vi "(FPGA)_PIDXYZ_laserPID)_COMtemp2.vi"() -> ()   [LabVIEW 2018]
doc: "This VI will read single point values from 4 channels of a R Series board at a specified rate."
uses:
  <vilib>/rvi/Emulation/niFpgaGetClockAttributes.vi
  <vilib>/rvi/Emulation/niFpgaSctlEmulationGetInTimedLoop.vi
  <vilib>/rvi/Emulation/niFpgaEmulationReportErrorSimple.vi
  <vilib>/rvi/eio/common/nirviEmuTemplateMethod_errors.vi
  <vilib>/rvi/Emulation/niFpgaProcessEmulError.vi
  <vilib>/rvi/Emulation/niFpgaCriticalErrorInLSC.vi
  <vilib>/rvi/Memory/Memory_Emulation/nirvimemoryFastEmulation.vi
  <vilib>/rvi/Memory/Memory_Emulation/nirvimemoryEmulation.vi
  <vilib>/rvi/Emulation/niFpgaEmulationIsFPGAContextNoSignature.vi
  <vilib>/rvi/DataTransferAndStorage/Container/Common/niFpgaContainerGetUniqueNameForEmu.vi
  <vilib>/rvi/errors/nirviReportUnexpectedCaseInternalError (U32).vi
  <vilib>/rvi/Memory/Memory_Emulation/niFpgaMemoryEmulationCacheClearOnFirstRun.vi
  <vilib>/rvi/Memory/Memory_Emulation/nirvimemoryEmulationManagerCache_MakeExclusive.vi
  <vilib>/rvi/Memory/Memory_Emulation/niFpgaMemoryEmulationValidateCache.vi
  <vilib>/rvi/Memory/Memory_Emulation/nirvimemoryEmulationManagerCache_InsertValue.vi
  <vilib>/Utility/error.llb/Clear Errors.vi
  <vilib>/rvi/Memory/Memory_Emulation/nirvimemoryEmulationManagerCache_ReleaseExclusive.vi
  <vilib>/rvi/Memory/Memory_Emulation/nirvimemoryEmulationManagerCache_GetValue.vi
  <vilib>/rvi/Memory/Memory_Emulation/nirvimemoryEmulationManagerCache_SetValue.vi
  <vilib>/rvi/Emulation/niFpgaSctlEmulationResourceMgr.vi
  <vilib>/eio/EIONode/EIONode.xnode
  <vilib>/rvi/DataTransferAndStorage/Container/XNode/niFpgaContainer.xnode
  <vilib>/rvi/FXPMathLib/FxpInterpret/XNode/nifxpmath_Interpret.xnode
panel:
  out "accum out z2":fxp<+/-,37,37>
  out "accurm reset z2":bool
  out "accum out z1":fxp<+/-,37,37>
  out "accum reset z1":bool
  in  "Reset x accum":bool
  in  "Reset y accum":bool
  in  "Reset z accum":bool
  out "master y":bool
  out "master x":bool
  in  "No_integral_gain":bool=TRUE
  in  "Y_emergency_threshould":i16
  in  "X_emergency_threshould":i16
  in  "Big Number":sgl
  in  "Amplitude_sine_EOM":sgl
  in  "eom sine frequency (periods/tick)":fxp<+,32,0>=0.0002500000409781933
  in  "pz?":bool
  out "pg Z mod":fxp<+/-,24,12>
  in  "pg Z":fxp<+/-,24,12>
  in  "amplitude":i16=8192
  in  "offset":i16=8192
  out "Trigger for COM out":i16 caption="square wave out"
  out "dgz mod":fxp<+/-,24,12>
  in  "activate COMz":bool
  in  "dg Z":fxp<+/-,24,12>
  in  "activate COMy":bool
  out "dgy mod":fxp<+/-,24,12>
  in  "dg Y":fxp<+/-,24,12>
  out "dgx mod":fxp<+/-,24,12>
  in  "activate COMx":bool
  in  "dg X":fxp<+/-,24,12>
  in  "duty cycle (periods)":fxp<+,32,0>=0.5
  in  "frequency (periods/tick)":fxp<+,32,0>=0.00390625
  in  "final filter coeff X before":i32[](array[numeric])=[-955995012, 2025731616, 1001305, -1023351008, 2092954700, 1034533]
  in  "final filter coeff X":i32[](array[numeric])=[-955995012, 2025731616, 1001305, -1023351008, 2092954700, 1034533]
  in  "final filter coeff Y before":i32[](array[numeric])=[-955995012, 2025731616, 1001305, -1023351008, 2092954700, 1034533]
  in  "final filter coeff Y":i32[](array[numeric])=[-955995012, 2025731616, 1001305, -1023351008, 2092954700, 1034533]
  in  "final filter coeff Z":i32[](array[numeric])=[-955995012, 2025731616, 1001305, -1023351008, 2092954700, 1034533]
  in  "final filter coeff Z before":i32[](array[numeric])=[-955995012, 2025731616, 1001305, -1023351008, 2092954700, 1034533]
  in  "LP Coeff Z before":i32[](array[numeric])=[1008310688, 32715568]
  in  "LP Coeff Z":i32[](array[numeric])=[1008310688, 32715568]
  in  "LP Coeff X":i32[](array[numeric])=[1008310688, 32715568]
  in  "LP Coeff X before":i32[](array[numeric])=[1008310688, 32715568]
  in  "LP Coeff Y before":i32[](array[numeric])=[1008310688, 32715568]
  in  "LP Coeff Y":i32[](array[numeric])=[1008310688, 32715568]
  in  "Upper lim Z before":fxp<+/-,16,16>
  in  "Lower lim Z before":fxp<+/-,16,16>
  in  "Upper lim Y before":fxp<+/-,16,16>
  in  "Lower lim Y before":fxp<+/-,16,16>
  in  "Upper lim X before":fxp<+/-,16,16>
  in  "Lower lim X before":fxp<+/-,16,16>
  in  "HP coeff band X before":i32[](array[numeric])=[-850883994, 1909449570, 958518847, -975456236, 2033039520, 1020559395]
  in  "LP Coeff band X before":i32[](array[numeric])=[-955995012, 2025731616, 1001305, -1023351008, 2092954700, 1034533]
  in  "LP Coeff band X":i32[](array[numeric])=[-955995012, 2025731616, 1001305, -1023351008, 2092954700, 1034533]
  in  "HP Coeff band X":i32[](array[numeric])=[-850883994, 1909449570, 958518847, -975456236, 2033039520, 1020559395]
  in  "dg band X before":fxp<+/-,24,12>
  in  "dg band X":fxp<+/-,24,12>
  in  "HP Coeff X before":i32[](array[numeric])=[946630756, 1010186290]
  in  "HP Coeff X":i32[](array[numeric])=[946630756, 1010186290]
  in  "Use X PID before":bool
  out "AI X before chamber plot":i16
  in  "X before Setpoint":i16
  out "tot_fb X plot":i16
  out "fb X before chamber plot":i16
  in  "DC offset X":i16
  in  "pg X before":fxp<+/-,24,12>
  in  "ig X before":fxp<+/-,24,-4>
  in  "dg X before":fxp<+/-,24,12>
  out "fb X plot":i16
  in  "ig X":fxp<+/-,24,-4>
  in  "Lower lim X":fxp<+/-,16,16>
  in  "Upper lim X":fxp<+/-,16,16>
  in  "pg X":fxp<+/-,24,12>
  out "AI X plot":i16
  in  "X Setpoint":i16
  in  "HP coeff band Y before":i32[](array[numeric])=[-850883994, 1909449570, 958518847, -975456236, 2033039520, 1020559395]
  in  "LP Coeff band Y before":i32[](array[numeric])=[-955995012, 2025731616, 1001305, -1023351008, 2092954700, 1034533]
  in  "LP Coeff band Y":i32[](array[numeric])=[-955995012, 2025731616, 1001305, -1023351008, 2092954700, 1034533]
  in  "HP Coeff band Y":i32[](array[numeric])=[-850883994, 1909449570, 958518847, -975456236, 2033039520, 1020559395]
  in  "dg band Y before":fxp<+/-,24,12>
  in  "dg band Y":fxp<+/-,24,12>
  in  "HP Coeff Y before":i32[](array[numeric])=[946630756, 1010186290]
  in  "HP Coeff Y":i32[](array[numeric])=[946630756, 1010186290]
  in  "Use Y PID before":bool
  out "AI Y before chamber plot":i16
  in  "Y before Setpoint":i16
  out "tot_fb Y plot":i16
  out "fb Y before chamber plot":i16
  in  "DC offset Y":i16
  in  "pg Y before":fxp<+/-,24,12>
  in  "ig Y before":fxp<+/-,24,-4>
  in  "dg Y before":fxp<+/-,24,12>
  out "fb Y plot":i16
  in  "ig Y":fxp<+/-,24,-4>
  in  "Lower lim Y":fxp<+/-,16,16>
  in  "Upper lim Y":fxp<+/-,16,16>
  in  "pg Y":fxp<+/-,24,12>
  out "AI Y plot":i16
  in  "Y Setpoint":i16
  in  "EOM_offset":i16
  in  "EOM_seed":u32=4294967295 caption="seed"
  in  "EOM reset":bool caption="reset"
  in  "EOM_threshold":i16
  in  "EOM_amplitude":i16
  in  "HP coeff band Z before":i32[](array[numeric])=[-850883994, 1909449570, 958518847, -975456236, 2033039520, 1020559395]
  in  "LP Coeff band Z before":i32[](array[numeric])=[-955995012, 2025731616, 1001305, -1023351008, 2092954700, 1034533]
  in  "LP Coeff band Z":i32[](array[numeric])=[-955995012, 2025731616, 1001305, -1023351008, 2092954700, 1034533]
  in  "HP Coeff band Z":i32[](array[numeric])=[-850883994, 1909449570, 958518847, -975456236, 2033039520, 1020559395]
  in  "dg band Z before":fxp<+/-,24,12>
  in  "dg band Z":fxp<+/-,24,12>
  in  "data_buffer3":i16
  in  "Arb gain (ch2)":fxp<+/-,24,12>=0.5 caption="RMS"
  in  "HP Coeff Z before":i32[](array[numeric])=[946630756, 1010186290]
  in  "HP Coeff Z":i32[](array[numeric])=[946630756, 1010186290]
  in  "Use Z PID before":bool
  out "AI Z before chamber plot":i16
  in  "Z before Setpoint":i16
  out "tot_fb Z plot":i16
  out "fb Z before chamber plot":i16
  in  "DC offset Z":i16
  in  "pg Z before":fxp<+/-,24,12>
  in  "ig Z before":fxp<+/-,24,-4>
  in  "dg Z before":fxp<+/-,24,12>
  out "fb Z plot":i16
  in  "ig Z":fxp<+/-,24,-4>
  out "written_address":u32
  in  "ready_to_write":bool
  in  "Arb steps per cycle":u16
  in  "data_buffer2":i16
  in  "data_buffer_1":i16
  in  "write_address":u16
  in  "Arb gain (ch1)":fxp<+/-,24,12>=0.5 caption="RMS"
  in  "Arb gain (ch0)":fxp<+/-,24,12>=0.5 caption="RMS"
  in  "Lower lim Z":fxp<+/-,16,16>
  in  "Upper lim Z":fxp<+/-,16,16>
  out "AI Z plot":i16
  in  "Z Setpoint":i16
  in  "Count(uSec)":u32
  out "FPGA Error Out":errorcluster
  in  "Stop":bool
  # "test"
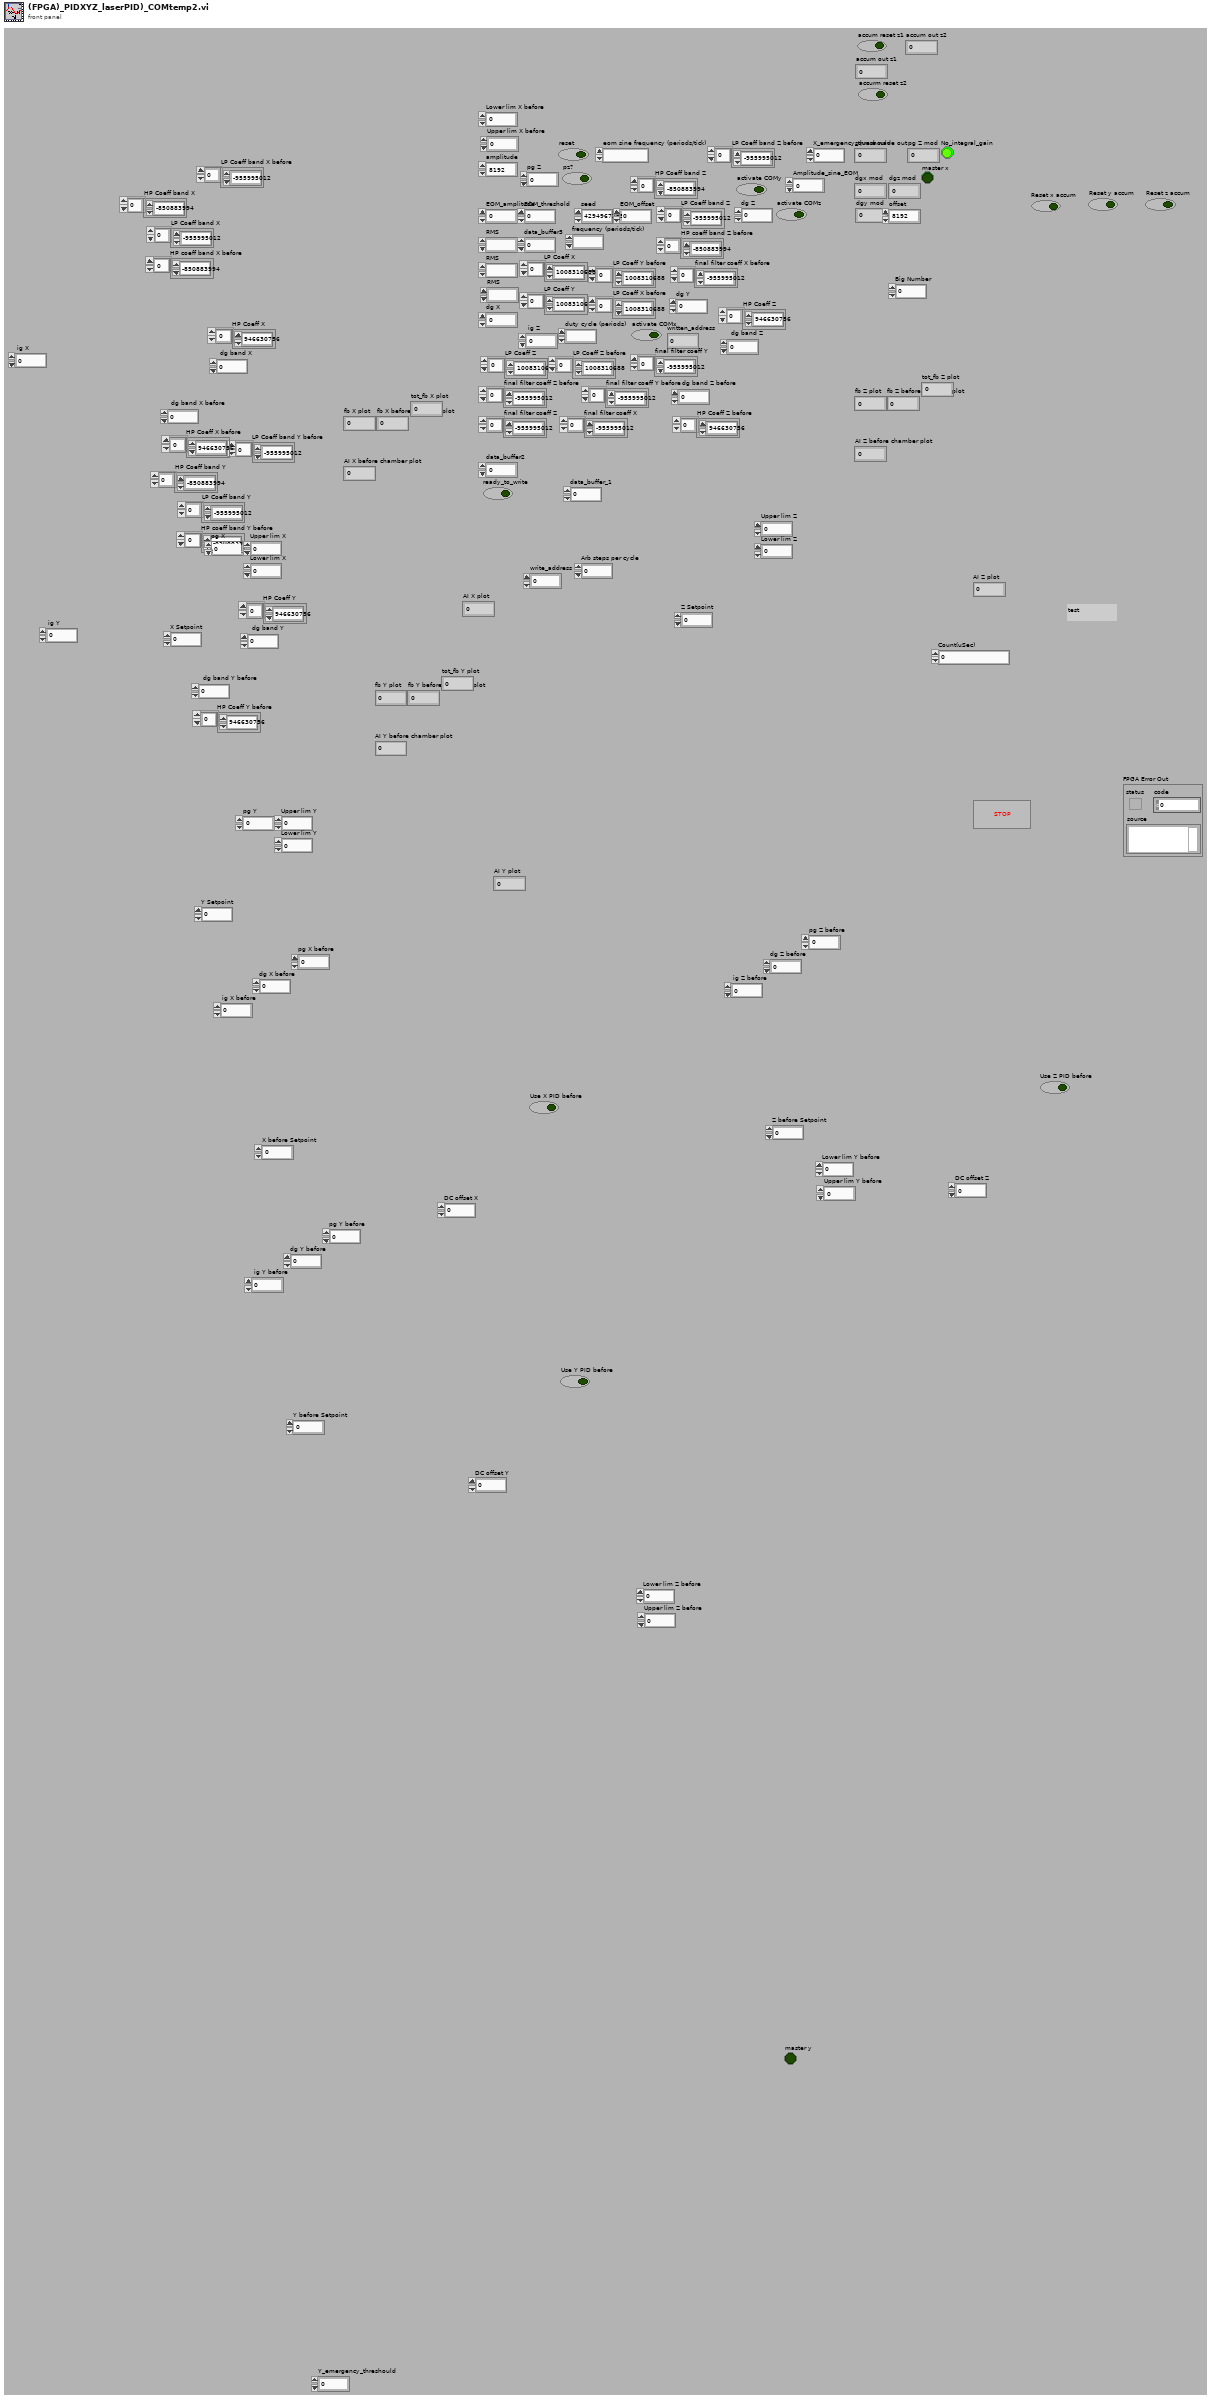
[diagram p1: front panel]
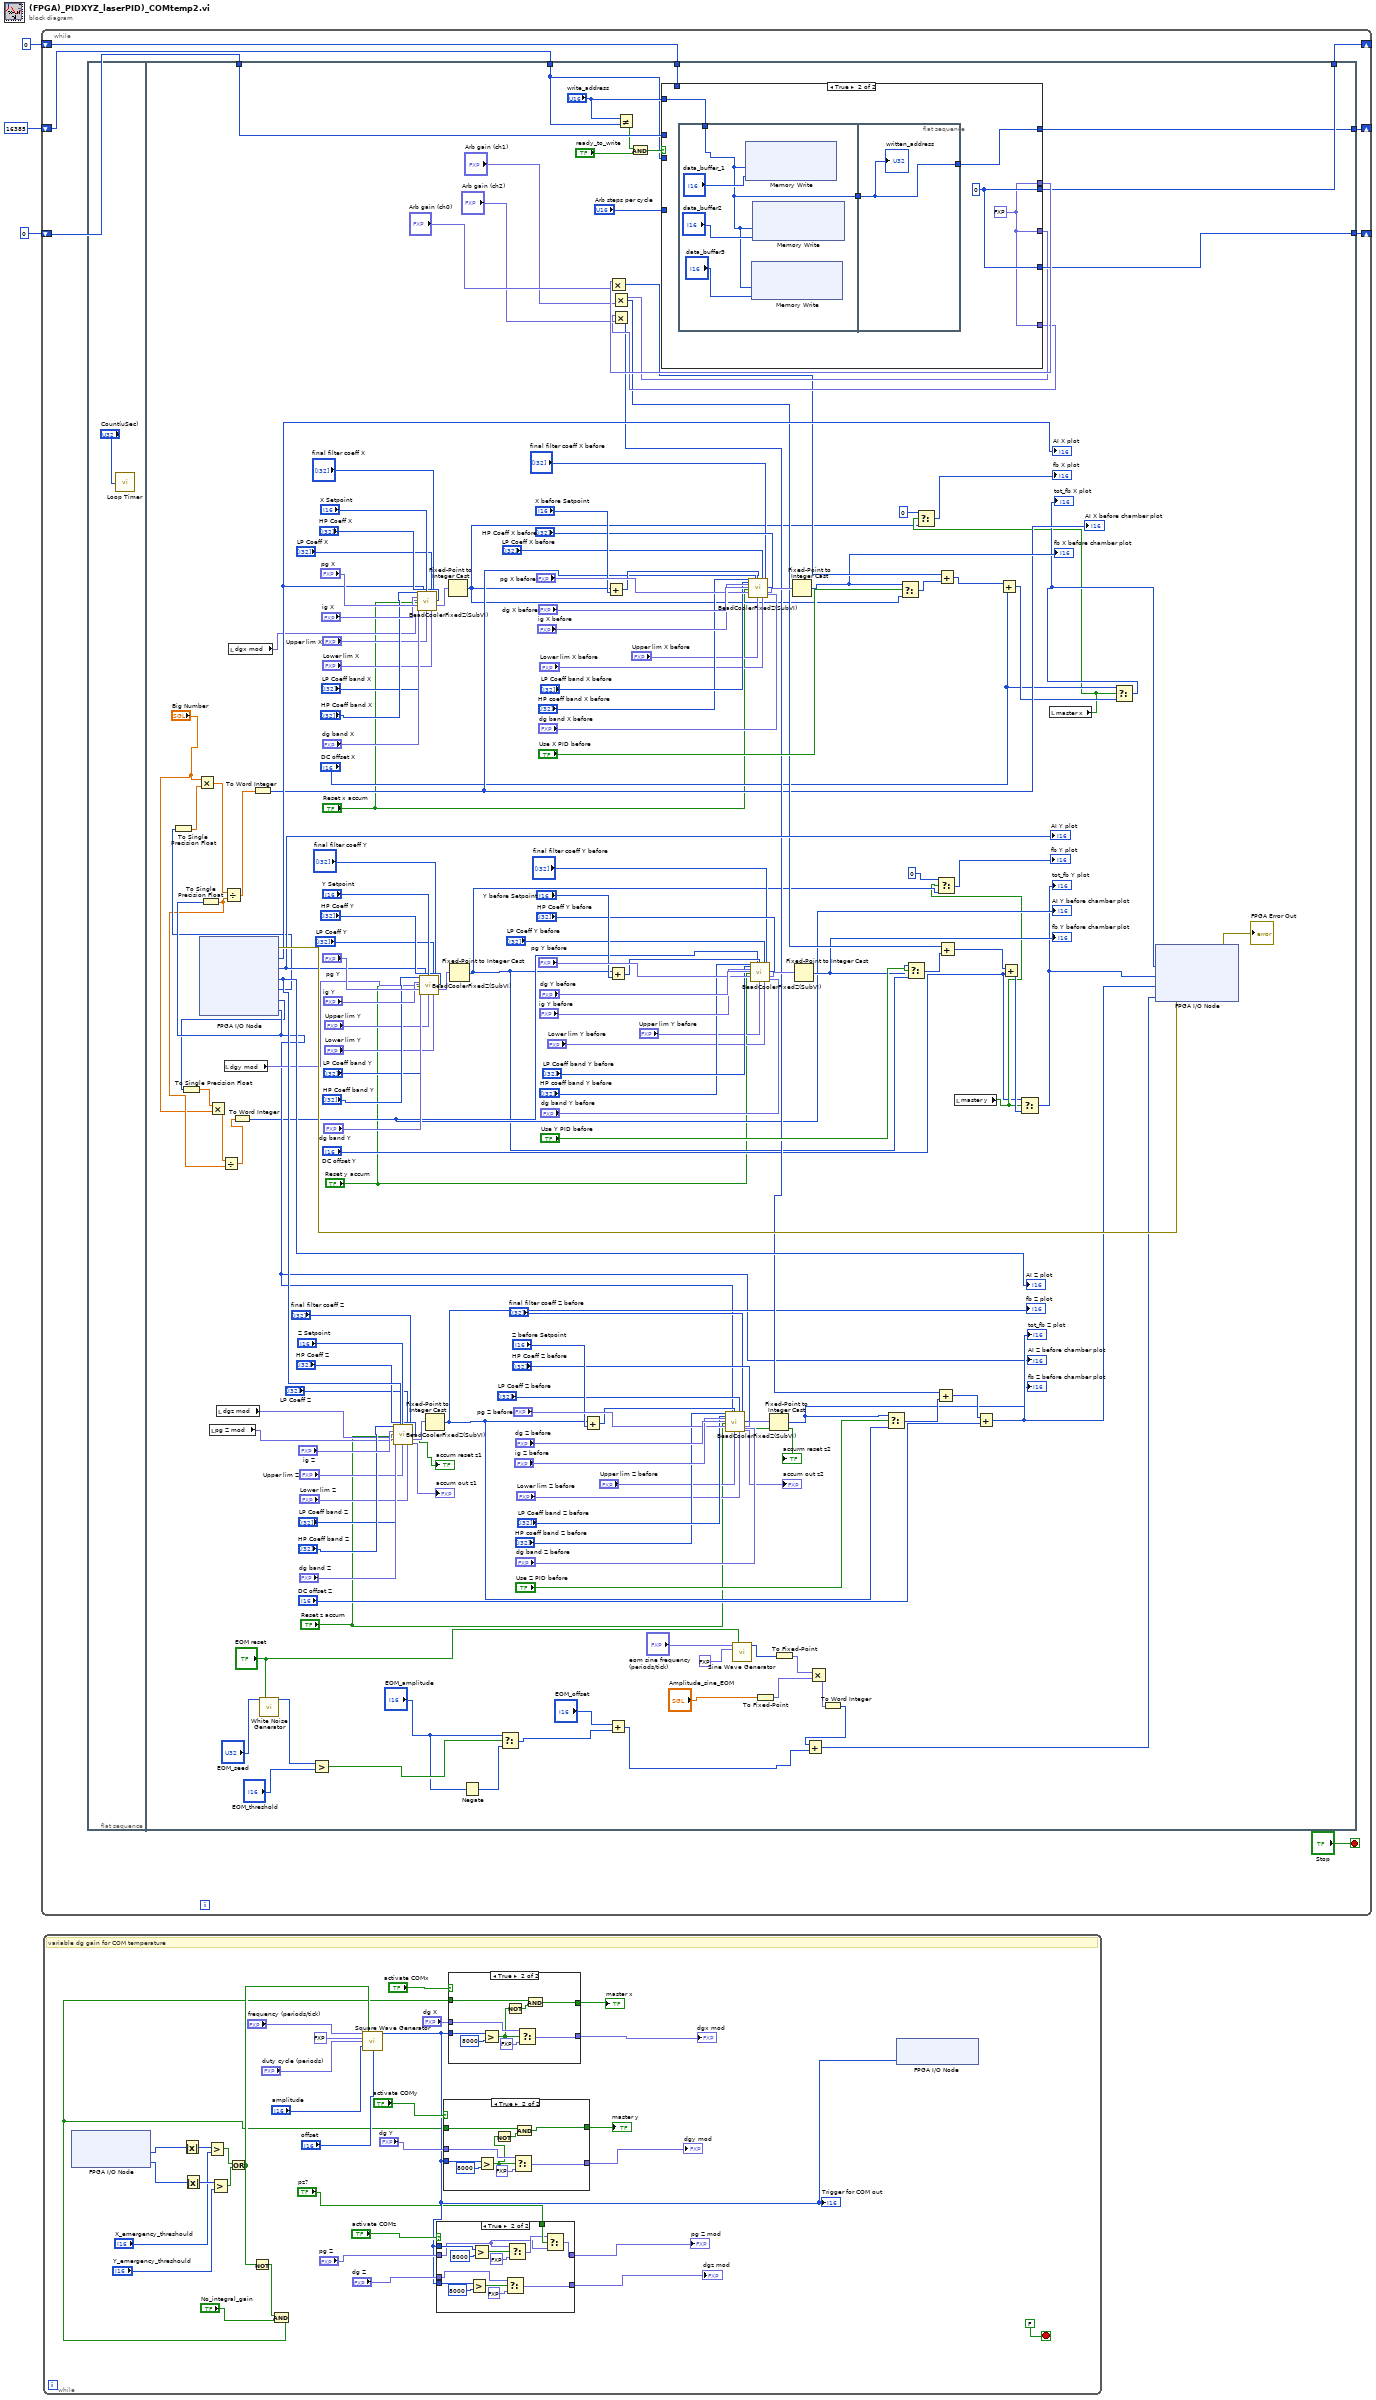
[diagram p0: block diagram]
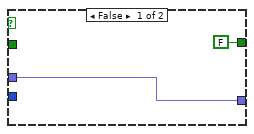
[diagram p3: hidden frame]
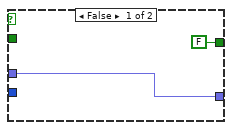
[diagram p4: hidden frame]
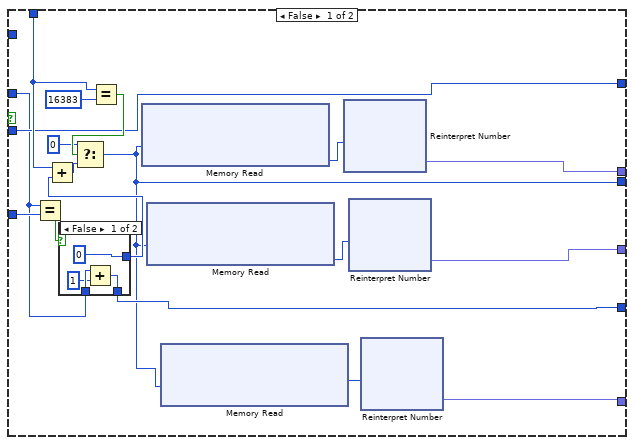
[diagram p5: hidden frame]
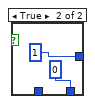
[diagram p6: hidden frame]
diagram:
  n1 = while {
    shift-right: [w9] -> _
    shift-left: u16 0 ("t") -> [w8]
    shift-right: [w7] -> _
    shift-left: u16 0 ("t") -> [w4]
    shift-right: [w6] -> _
    shift-left: u32 16385 ("write_address") -> [w5]
    stop <- "Stop" stop-if-true
    n2 = flat-sequence {
      tunnel: [w180] -> w9
      tunnel: w8 -> [w179]
      tunnel: [w177] -> w7
      tunnel: w4 -> [w176]
      tunnel: [w175] -> w6
      tunnel: w5 -> [w168]
      frame #0 {
        n3 = call "Loop Timer"("Count(uSec)"="Count(uSec)") -> ()  [unwired: 1 out]
      }
      frame #1 {
        n4 = xnode "FPGA I/O Node"() -> ("error out"=w185:errorcluster, "Connector0/AI0"=w92:i16, "Connector0/AI1"=w114:i16, "Connector0/AI2"=w166:i16, "Connector0/AI3"=w40:i16, "Connector0/AI4"=w39:i16, "Connector0/AI5"=w44:i16)  [unwired: 7 in, 6 out]
        "AI Z plot" <- w166
        "AI Z before chamber plot" <- w44
        "AI Y plot" <- w114
        "AI X plot" <- w92
        n5 = To Single Precision Float(number=w40) -> (single precision float=w43:sgl)
        n6 = To Single Precision Float(number=w39) -> (single precision float=w38:sgl)
        n7 = Multiply(x="Big Number", y=w43) -> (x*y=w42:sgl)
        n8 = To Single Precision Float(number=w44) -> (single precision float=w36:sgl)
        n9 = Multiply(x=w38, y="Big Number") -> (x*y=w37:sgl)
        n10 = local read "pg Z mod"() -> (w57:fxp<+/-,24,12>)
        n11 = local read "dgz mod"() -> (w58:fxp<+/-,24,12>)
        n12 = Divide(x=w37, y=w36) -> (x/y=w35:sgl)
        n13 = Divide(x=w42, y=w36) -> (x/y=w41:sgl)
        n14 = local read "dgy mod"() -> (w59:fxp<+/-,24,12>)
        n15 = local read "dgx mod"() -> (w60:fxp<+/-,24,12>)
        n16 = To Word Integer(number=w35) -> (16bit integer=w34:i16)
        "AI Y before chamber plot" <- w34
        n17 = To Word Integer(number=w41) -> (16bit integer=w45:i16)
        "AI X before chamber plot" <- w45
        n18 = call "White Noise Generator"("seed"="EOM_seed", "reset"="EOM reset") -> ("white noise out"=w145:i16)  [unwired: 13 in]
        n19 = Greater?(x=w145, y="EOM_threshold") -> (0:w143:bool)
        n20 = call "BeadCoolerFixedZ(SubVI).vi"("hp coeff band"="HP Coeff band Z", "lp coeff band"="LP Coeff band Z", "ig"="ig Z", "dg"=w58, "load (F)"="Reset z accum", "pg"=w57, "dg band"="dg band Z", "AI0"=w166, "Dc Pos"="Z Setpoint", "Upper lim"="Upper lim Z", "lp coeff"="LP Coeff Z", "Lower lim"="Lower lim Z", "final filter coeff"="final filter coeff Z", "hp coeff"="HP Coeff Z") -> ("Output"=w155:fxp<+/-,16,16>, "accurm reset"=→"accum reset z1":bool, "accum out"=→"accum out z1":fxp<+/-,37,37>)  [unwired: 11 in]
        n21 = call "BeadCoolerFixedZ(SubVI).vi"("hp coeff band"="HP Coeff band X", "lp coeff band"="LP Coeff band X", "ig"="ig X", "dg"=w60, "load (F)"="Reset x accum", "pg"="pg X", "dg band"="dg band X", "AI0"=w92, "Dc Pos"="X Setpoint", "Upper lim"="Upper lim X", "lp coeff"="LP Coeff X", "Lower lim"="Lower lim X", "final filter coeff"="final filter coeff X", "hp coeff"="HP Coeff X") -> ("Output"=w102:fxp<+/-,16,16>)  [unwired: 11 in, 2 out]
        n22 = call "BeadCoolerFixedZ(SubVI).vi"("hp coeff band"="HP Coeff band Y", "lp coeff band"="LP Coeff band Y", "ig"="ig Y", "dg"=w59, "load (F)"="Reset y accum", "pg"="pg Y", "dg band"="dg band Y", "AI0"=w114, "Dc Pos"="Y Setpoint", "Upper lim"="Upper lim Y", "lp coeff"="LP Coeff Y", "Lower lim"="Lower lim Y", "final filter coeff"="final filter coeff Y", "hp coeff"="HP Coeff Y") -> ("Output"=w124:fxp<+/-,16,16>)  [unwired: 11 in, 2 out]
        n23 = Fixed-Point to Integer Cast(1:w155) -> (0:w70:i16)
        "fb Z plot" <- w70
        n24 = Fixed-Point to Integer Cast(1:w102) -> (0:w20:i16)
        n25 = Fixed-Point to Integer Cast(1:w124) -> (0:w28:i16)
        n26 = Negate(x="EOM_amplitude") -> (-x=w141:i16)
        n27 = Select(t="EOM_amplitude", s=w143, f=w141) -> (s? t:f=w139:i16)
        n28 = Add(x=w70, y="Z before Setpoint") -> (x+y=w154:i16)
        n29 = Add(x=w20, y="X before Setpoint") -> (x+y=w101:i16)
        n30 = Add(x=w28, y="Y before Setpoint") -> (x+y=w123:i16)
        n31 = Add(x="EOM_offset", y=w139) -> (x+y=w48:i16)
        n32 = Not Equal?(x="write_address", y=w168) -> (x != y?=w172:bool)
        n33 = And(x=w172, y="ready_to_write") -> (x .and. y?=w173:bool)
        n34 = case shown="True" w173 {
          tunnel: [w202 w210] -> w182
          tunnel: [w187 w214] -> w180
          tunnel: w179 -> [w195 _]
          tunnel: [w196 w210] -> w170
          tunnel: "Arb steps per cycle" -> [w194 _]
          tunnel: [w189 w214] -> w177
          tunnel: w176 -> [w190 _]
          tunnel: [w193 w212] -> w175
          tunnel: w168 -> [w193 _]
          tunnel: "write_address" -> [_ w211]
          tunnel: [w186 w210] -> w152
          frame False {
            n35 = Equal?(x=w190, y=w194) -> (x = y?=w192:bool)
            n36 = case shown="False" w192 {
              tunnel: [u16 0 ("y") u16 1 ("y")] -> w191
              tunnel: w190 -> [w206 _]
              tunnel: [w204 u16 0] -> w189
              frame False {
                n37 = Add(x=w206, y=u16 1) -> (x+y=w204:u16)
              }
              frame True {
              }
            }
            n38 = Add(x=w195, y=w191) -> (x+y=w198:u16)
            n39 = Equal?(x=w195, y=u16 16383) -> (x = y?=w200:bool)
            n40 = Select(t=u16 0, s=w200, f=w198) -> (s? t:f=w187:u16)
            n41 = xnode ("Memory Read")("Address"=w187) -> ("Data"=w203:i16)  [unwired: 1 in, 1 out]
            n42 = xnode ("Memory Read")("Address"=w187) -> ("Data"=w197:i16)  [unwired: 1 in, 1 out]
            n43 = xnode ("Memory Read")("Address"=w187) -> ("Data"=w188:i16)  [unwired: 1 in, 1 out]
            n44 = xnode "Reinterpret Number"("x"=w203) -> ("y"=w202:fxp<+/-,16,16>)
            n45 = xnode "Reinterpret Number"("x"=w197) -> ("y"=w196:fxp<+/-,16,16>)
            n46 = xnode "Reinterpret Number"("x"=w188) -> ("y"=w186:fxp<+/-,16,16>)
          }
          frame True {
            w214 = u16 0
            w210 = fxp<+/-,16,16> 0.0 ("y")
            n47 = flat-sequence {
              tunnel: [w216] -> w213
              tunnel: w211 -> [w216]
              tunnel: w213 -> [w219]
              tunnel: [w219] -> w212
              frame #0 {
                n48 = xnode ("Memory Write")("Address"=w216, "Data"="data_buffer_1") -> ()  [unwired: 1 in, 1 out]
                n49 = xnode ("Memory Write")("Address"=w216, "Data"="data_buffer3") -> ()  [unwired: 1 in, 1 out]
                n50 = xnode ("Memory Write")("Address"=w216, "Data"="data_buffer2") -> ()  [unwired: 1 in, 1 out]
              }
              frame #1 {
                "written_address" <- w219
              }
            }
          }
        }
        n51 = Multiply(x=w182, y="Arb gain (ch0)") -> (x*y=w73:i16)
        n52 = Multiply(x=w170, y="Arb gain (ch1)") -> (x*y=w72:i16)
        n53 = Multiply(x=w152, y="Arb gain (ch2)") -> (x*y=w71:i16)
        n54 = call "BeadCoolerFixedZ(SubVI).vi"("hp coeff band"="HP coeff band Z before", "lp coeff band"="LP Coeff band Z before", "ig"="ig Z before", "dg"="dg Z before", "load (F)"="Reset z accum", "pg"="pg Z before", "dg band"="dg band Z before", "AI0"=w44, "Dc Pos"=w154, "Upper lim"="Upper lim Z before", "lp coeff"="LP Coeff Z before", "Lower lim"="Lower lim Z before", "final filter coeff"="final filter coeff Z before", "hp coeff"="HP Coeff Z before") -> ("Output"=w162:fxp<+/-,16,16>, "accurm reset"=→"accurm reset z2":bool, "accum out"=→"accum out z2":fxp<+/-,37,37>)  [unwired: 11 in]
        n55 = call "Sine Wave Generator"("frequency (periods/tick)"="eom sine frequency (periods/tick)", "reset"="EOM reset", "phase offset (periods)"=fxp<+,32,0> 0.0) -> ("sine out"=w54:i16)  [unwired: 12 in]
        n56 = call "BeadCoolerFixedZ(SubVI).vi"("hp coeff band"="HP coeff band X before", "lp coeff band"="LP Coeff band X before", "ig"="ig X before", "dg"="dg X before", "load (F)"="Reset x accum", "pg"="pg X before", "dg band"="dg band X before", "AI0"=w45, "Dc Pos"=w101, "Upper lim"="Upper lim X before", "lp coeff"="LP Coeff X before", "Lower lim"="Lower lim X before", "final filter coeff"="final filter coeff X before", "hp coeff"="HP Coeff X before") -> ("Output"=w107:fxp<+/-,16,16>)  [unwired: 11 in, 2 out]
        n57 = call "BeadCoolerFixedZ(SubVI).vi"("hp coeff band"="HP coeff band Y before", "lp coeff band"="LP Coeff band Y before", "ig"="ig Y before", "dg"="dg Y before", "load (F)"="Reset y accum", "pg"="pg Y before", "dg band"="dg band Y before", "AI0"=w34, "Dc Pos"=w123, "Upper lim"="Upper lim Y before", "lp coeff"="LP Coeff Y before", "Lower lim"="Lower lim Y before", "final filter coeff"="final filter coeff Y before", "hp coeff"="HP Coeff Y before") -> ("Output"=w129:fxp<+/-,16,16>)  [unwired: 11 in, 2 out]
        n58 = To Fixed-Point(number="Amplitude_sine_EOM") -> (fixed-point=w52:fxp<+/-,32,16>)  [unwired: 1 in]
        n59 = Fixed-Point to Integer Cast(1:w162) -> (0:w61:i16)
        "fb Z before chamber plot" <- w61
        n60 = To Fixed-Point(number=w54) -> (fixed-point=w53:fxp<+/-,16,16>)  [unwired: 1 in]
        n61 = Fixed-Point to Integer Cast(1:w107) -> (0:w67:i16)
        "fb X before chamber plot" <- w67
        n62 = Fixed-Point to Integer Cast(1:w129) -> (0:w64:i16)
        "fb Y before chamber plot" <- w64
        n63 = Multiply(x=w53, y=w52) -> (x*y=w51:fxp<+/-,48,32>)
        n64 = To Word Integer(number=w51) -> (16bit integer=w49:i16)
        n65 = Add(x=w49, y=w48) -> (x+y=w47:i16)
        n66 = Select(t=w61, s="Use Z PID before", f=w70) -> (s? t:f=w63:i16)
        n67 = Select(t=w67, s="Use X PID before", f=w20) -> (s? t:f=w69:i16)
        n68 = Select(t=w64, s="Use Y PID before", f=w28) -> (s? t:f=w66:i16)
        n69 = Add(x=w71, y=w63) -> (x+y=w62:i16)
        n70 = Add(x=w73, y=w69) -> (x+y=w68:i16)
        n71 = Add(x=w72, y=w66) -> (x+y=w65:i16)
        n72 = local read "master y"() -> (w27:bool)
        n73 = Select(t=i16 0, s=w27, f=w28) -> (s? t:f=→"fb Y plot":i16)
        n74 = Add(x=w62, y="DC offset Z") -> (x+y=w158:i16)
        "tot_fb Z plot" <- w158
        n75 = Add(x=w68, y="DC offset X") -> (x+y=w25:i16)
        n76 = Add(x=w65, y="DC offset Y") -> (x+y=w32:i16)
        n77 = Select(t="DC offset Y", s=w27, f=w32) -> (s? t:f=w31:i16)
        "tot_fb Y plot" <- w31
        n78 = local read "master x"() -> (w22:bool)
        n79 = Select(t=i16 0, s=w22, f=w20) -> (s? t:f=→"fb X plot":i16)
        n80 = Select(t="DC offset X", s=w22, f=w25) -> (s? t:f=w24:i16)
        "tot_fb X plot" <- w24
        n81 = xnode "FPGA I/O Node"("error in"=w185, "Connector0/AO0"=w24, "Connector0/AO1"=w31, "Connector0/AO2"=w158, "Connector0/AO3"=w47) -> ("error out"=→"FPGA Error Out":errorcluster)  [unwired: 4 in, 4 out]
      }
    }
  }
  n82 = while {
    stop <- FALSE stop-if-true
    # "variable dg gain for COM temperature"
    n83 = xnode "FPGA I/O Node"() -> ("Connector0/AI0"=w233:i16, "Connector0/AI1"=w232:i16)  [unwired: 3 in, 3 out]
    n84 = Absolute Value(x=w233) -> (abs(x)=w231:i16)
    n85 = Absolute Value(x=w232) -> (abs(x)=w230:i16)
    n86 = Greater?(x=w231, y="X_emergency_threshould") -> (0:w227:bool)
    n87 = Greater?(x=w230, y="Y_emergency_threshould") -> (0:w226:bool)
    n88 = Or(x=w227, y=w226) -> (x .or. y?=w225:bool)
    n89 = Not(x=w225) -> (.not. x?=w224:bool)
    n90 = And(x=w224, y="No_integral_gain") -> (x .and. y?=w222:bool)
    n91 = call "Square Wave Generator"("frequency (periods/tick)"="frequency (periods/tick)", "reset"=w225, "phase offset (periods)"=fxp<+,32,0> 0.0, "duty cycle (periods)"="duty cycle (periods)", "amplitude"="amplitude", "offset"="offset") -> ("square wave out"=w235:i16)  [unwired: 9 in]
    "Trigger for COM out" <- w235
    n92 = case shown="True" "activate COMz" {
      tunnel: [w254 w265] -> w238
      tunnel: w235 -> [_ w268]
      tunnel: "dg Z" -> [w254 w263]
      tunnel: "pg Z" -> [w253 w255]
      tunnel: [w253 w256] -> w236
      tunnel: w235 -> [_ w259]
      tunnel: "pz?" -> [_ w258]
      frame False {
      }
      frame True {
        n93 = Greater?(x=w268, y=i16 8000) -> (0:w266:bool)
        n94 = Greater?(x=w259, y=i16 8000) -> (0:w261:bool)
        n95 = Select(t=w263, s=w266, f=fxp<+/-,24,12> 0.0 ("y")) -> (s? t:f=w265:fxp<+/-,24,12>)
        n96 = Select(t=w255, s=w261, f=fxp<+/-,24,12> 0.0 ("y")) -> (s? t:f=w257:fxp<+/-,24,12>)
        n97 = Select(t=w257, s=w258, f=w255) -> (s? t:f=w256:fxp<+/-,24,12>)
      }
    }
    "dgz mod" <- w238
    "pg Z mod" <- w236
    n98 = case shown="True" "activate COMy" {
      tunnel: "dg Y" -> [w270 w276]
      tunnel: [w270 w277] -> w242
      tunnel: w235 -> [_ w279]
      tunnel: w222 -> [_ w273]
      tunnel: [FALSE w271] -> w220
      frame False {
      }
      frame True {
        n99 = Greater?(x=w279, y=i16 8000) -> (0:w272:bool)
        n100 = Not(x=w272) -> (.not. x?=w274:bool)
        n101 = Select(t=w276, s=w272, f=fxp<+/-,24,12> 0.0 ("y")) -> (s? t:f=w277:fxp<+/-,24,12>)
        n102 = And(x=w273, y=w274) -> (x .and. y?=w271:bool)
      }
    }
    "dgy mod" <- w242
    "master y" <- w220
    n103 = case shown="True" "activate COMx" {
      tunnel: "dg X" -> [w281 w287]
      tunnel: [w281 w288] -> w244
      tunnel: w235 -> [_ w290]
      tunnel: w222 -> [_ w283]
      tunnel: [FALSE w282] -> w221
      frame False {
      }
      frame True {
        n104 = Greater?(x=w290, y=i16 8000) -> (0:w285:bool)
        n105 = Not(x=w285) -> (.not. x?=w284:bool)
        n106 = Select(t=w287, s=w285, f=fxp<+/-,24,12> 0.0 ("y")) -> (s? t:f=w288:fxp<+/-,24,12>)
        n107 = And(x=w283, y=w284) -> (x .and. y?=w282:bool)
      }
    }
    "dgx mod" <- w244
    "master x" <- w221
    n108 = xnode "FPGA I/O Node"("Connector0/AO7"=w235) -> ()  [unwired: 2 in, 2 out]
  }
